vi "Software Update HCC Move DLL Data Folder to Archive.vi"(7 "Path Build List Sub":path, 8 "error in (no error)":errorcluster, 9 "folder names":string[](array[string]), 11 "Archive Target Folder":path) -> (0 "error out":errorcluster)   [LabVIEW 2016]
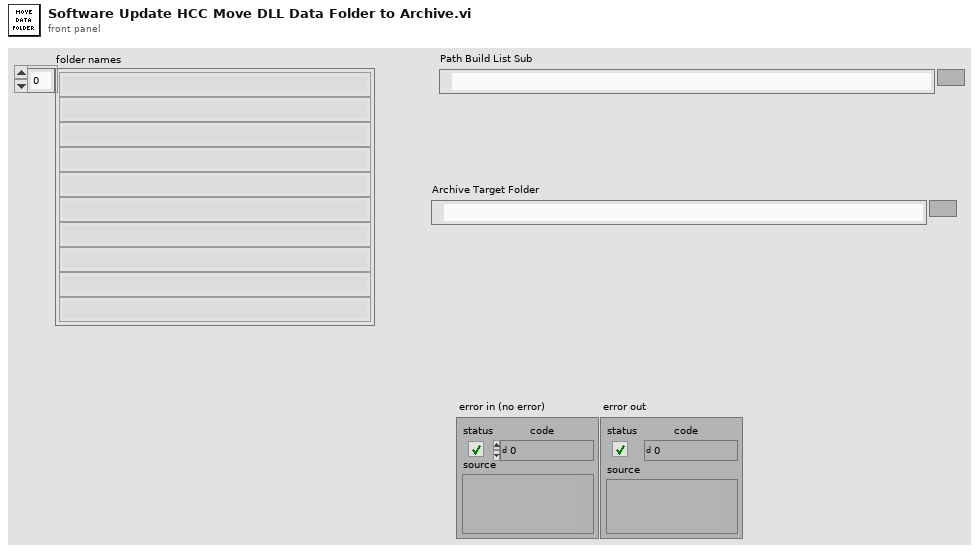
[diagram p1: front panel]
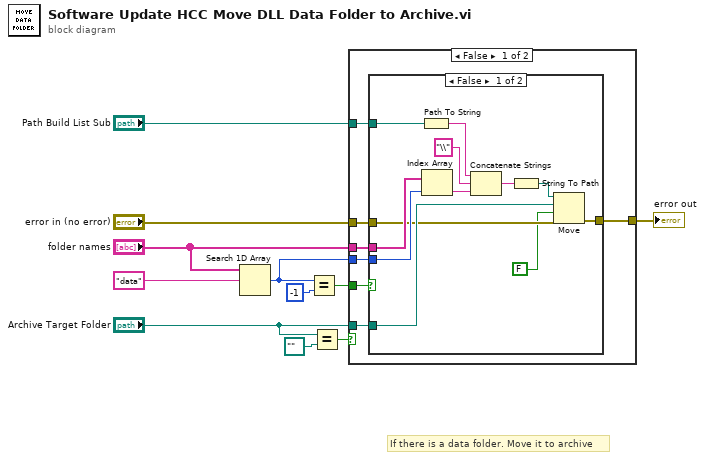
[diagram p0: block diagram]
diagram:
  # "If there is a data folder. Move it to archive"
  n1 = Search 1D Array(1D array="folder names", element="data") -> (index of element=w9:i32)  [unwired: 1 in]
  n2 = Equal?(x=w9, y=-1) -> (x = y?=w7:bool)
  n3 = Equal?(x="Archive Target Folder", y=path "") -> (x = y?=w3:bool)
  n4 = case shown="False" w3 {
    tunnel: "folder names" -> [w18 _]
    tunnel: w9 -> [w17 _]
    tunnel: w7 -> [w16 _]
    tunnel: "Path Build List Sub" -> [w15 _]
    tunnel: "Archive Target Folder" -> [w14 _]
    tunnel: "error in (no error)" -> [w13 w32]
    tunnel: [w12 w32] -> w1
    frame False {
      n5 = case shown="False" w16 {
        tunnel: w18 -> [w30 _]
        tunnel: w17 -> [w25 _]
        tunnel: w15 -> [w23 _]
        tunnel: w14 -> [w22 _]
        tunnel: w13 -> [w21 w31]
        tunnel: [w20 w31] -> w12
        frame False {
          n6 = Path To String(path=w23) -> (string=w29:string)
          n7 = Index Array(array=w30, index=w25) -> (element=w27:string)
          n8 = Concatenate Strings(w29, "\\" ("string"), w27) -> (w26:string)
          n9 = String To Path(string=w26) -> (path=w24:path)
          n10 = Move(source path=w24, error in=w21, 9:FALSE ("overwrite (F)"), 10:w22) -> (error out=w20:errorcluster)  [unwired: 1 in, 2 out]
        }
        frame True {
        }
      }
    }
    frame True {
    }
  }
  "error out" <- w1
